vi "Create.vi"(5 "Shutdown Timeout (ms)":u32=10000, 7 "Execution Timeout (ms)":u32=10000, 8 "error in (no error)":errorcluster, 10 "Pound":refnum<class "Pound.lvclass">, 11 "Name":string) -> (0 "error out":errorcluster, 3 "Watchdog":refnum<data-value>)   [LabVIEW 2017, in "Watchdog.lvclass"]
doc: "Create a watch dog reference."
uses:
  <vilib>/NI/Software Watchdog/Watchdog/Watchdog.lvclass
  <vilib>/NI/Software Watchdog/Pound/Pound.lvclass
  <vilib>/NI/Software Watchdog/Watchdog/Watchdog.lvclass/Watchdog.ctl
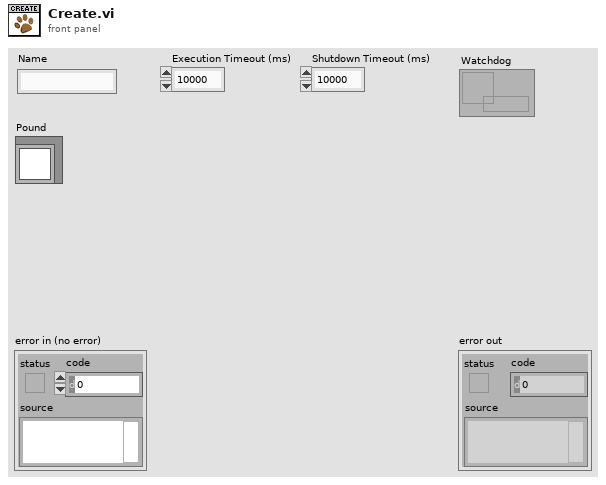
[diagram p1: front panel]
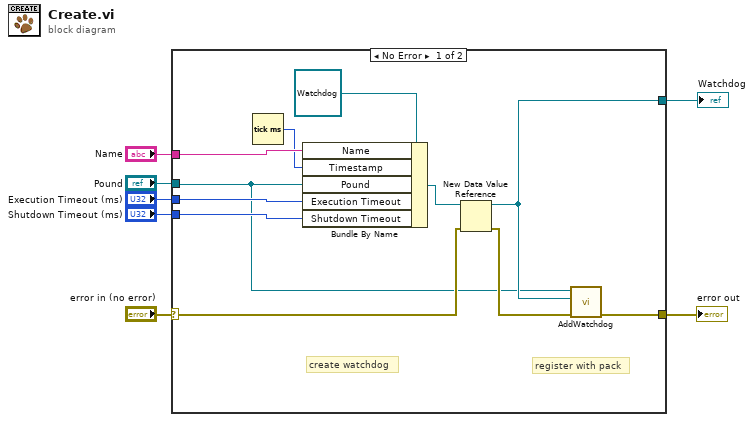
[diagram p0: block diagram]
diagram:
  n1 = case shown="No Error" "error in (no error)" {
    selector: "error in (no error)" -> [w17 w19]
    tunnel: [w12 w19] -> w6
    tunnel: [w11 _] -> w4
    tunnel: "Name" -> [w18 _]
    tunnel: "Pound" -> [w8 _]
    tunnel: "Execution Timeout (ms)" -> [w10 _]
    tunnel: "Shutdown Timeout (ms)" -> [w9 _]
    frame No Error {
      # "register with pack"
      # "create watchdog"
      n2 = Tick Count (ms)() -> (millisecond timer value=w16:u32)
      n3 = Bundle By Name(cluster=refnum<class "Watchdog.lvclass"> refnum ("Watchdog.lvclass"), "Name"=w18, "Timestamp"=w16, "Pound"=w8, "Execution Timeout"=w10, "Shutdown Timeout"=w9) -> (w15:refnum<class "Watchdog.lvclass">)
      n4 = New Data Value Reference(data value=w15, error in=w17) -> (data value reference=w11:refnum<data-value>, error out=w13:errorcluster)
      n5 = call <vilib>:"AddWatchdog.vi"("error in (no error)"=w13, "Watchdog"=w11, "Pound in"=w8) -> ("error out"=w12:errorcluster)  [unwired: 7 in, 1 out]
    }
    frame Error {
    }
  }
  "error out" <- w6
  "Watchdog" <- w4
